vi "navX Open.vi"(4 "Nav6Mode (YPR)":T2, 5 "I2C Bus":T9=enum."I2C MXP", 6 "Serial Port":T1, 7 "SPI Bus":T7=enum."SPI MXP", 8 "error in":errorcluster, 10 "Update Rate (4Hz-60Hz)":T20=50 min=4 max=60 step=1, 11 "navX Interface Protocol":T4) -> (0 "error out":errorcluster, 1 "Opened?":bool, 3 "navX Device TypeDef":T3={"navX Interface Protocol"=enum."SPI", "navX Interface Protocol TypeDefs"={"SPIDevRef"={"DevStatus"={"status"=FALSE, "code"=0, "source"=""}, "Handle"=0, "Controller"=enum."Controller 1", "SPI Bus"=enum."SPI On-Board, CS0"}, "I2CDevRef"={"DevStatus"={"status"=FALSE, "code"=0, "source"=""}, "Controller"=enum."Controller 1", "Device Address"=0, "Handle"=0, "I2C Bus"=enum."Invalid"}, "SerialPortRef"={"DevStatus"={"status"=FALSE, "code"=0, "source"=""}, "Serial Port Name"=""}}, "navX System Information"={"Board Information"={"WhoAmI (50 | 0x32)"=0, "Board Revision"=0, "Firmware Major Version"=0, "Firmware Minor Version"=0, "NAVX_BOARD_CAPABILITY"={"OMNIMOUNT"=FALSE, "YAW_RESET"=FALSE, "VEL_AND_DISP"=FALSE}, "NAVX_BOARD_YAW_AXIS"={"BOARD_YAW_AXIS_UP"=FALSE, "BOARD_YAW_AXIS"=0}}, "Status"={"Update Rate Hz"=0, "Accelerometer Full-Scale Range"=0, "Gyro Full-Scale Range"=0, "NAVX_OP_STATUS"=0, "NAVX_CAL_STATUS"=0, "NAVX_SELFTEST_STATUS"=0, "NAVX_SENSOR_STATUS"={"MOVING"=FALSE, "YAW_STABLE"=FALSE, "MAG_DISTURBANCE"=FALSE, "ALTITUDE_VALID"=FALSE, "SEALEVEL_PRESS_SET"=FALSE, "FUSED_HEADING_VALID"=FALSE}}, "Offsets"={"Yaw"=0.0, "Quat W"=0.0, "Quat X"=0.0, "Quat Y"=0.0, "Quat Z"=0.0}, "LastSampleTimestamp"=0.0, "LastSampleValid"=FALSE}, "navX Common Information"={"Update Rate (4Hz-60Hz)"=50, "refnum name"="", "error"={"status"=FALSE, "code"=0, "source"=""}, "LastFPGATimestamp"=0.0, "Reboot Detected"=FALSE}, "Serial Protocol Extra"={"Loop VI Refnum"=refnum, "Nav6Mode (YPR)"=enum."Raw"}} {"navX Common Information"."Update Rate (4Hz-60Hz)" min=4 max=60 step=1; "navX System Information"."Status"."NAVX_OP_STATUS" items=["INITIALIZING", "SELFTEST_IN_PROGRESS", "ERROR", "IMU_AUTOCAL_IN_PROGRESS", "NORMAL"]; "navX System Information"."Status"."NAVX_CAL_STATUS" items=["IMU_CAL_STATE_MASK"=3, "IMU_CAL_INPROGRESS"=0, "IMU_CAL_ACCUMULATE"=1, "IMU_CAL_COMPLETE"=2, "MAG_CAL_COMPLETE"=4, "BARO_CAL_COMPLETE"=8]; "navX System Information"."Status"."NAVX_SELFTEST_STATUS" items=["COMPLETE"=80, "GYRO_PASSED"=1, "ACCEL_PASSED"=2, "MAG_PASSED"=4, "BARO_PASSED"=8]; "navX Interface Protocol TypeDefs"."I2CDevRef"."Device Address" format="%.0x"})   [LabVIEW 2014, in "navX Library v1 (deprecated).lvlib"]
doc: "This VI is used to open the connection to a navX MXP unit over SPI or I2C."
uses:
  navX Library v1 (deprecated).lvlib
  TypeDefs/Value TypeDefs/navX Interface Protocol.ctl
  TypeDefs/Value TypeDefs/navX Update Rate.ctl
  <vilib>/Rock Robotics/SystemInterfaces/spilib/spi_bus.ctl
  <vilib>/Rock Robotics/SystemInterfaces/i2clib/i2c_bus.ctl
  TypeDefs/navX Device TypeDef.ctl
  <vilib>/Rock Robotics/WPI/SPI/WPI_SPIDevRef.ctl
  <vilib>/Rock Robotics/SystemInterfaces/Typedef/FPGA_TypedefDigitalModule.ctl
  <vilib>/Rock Robotics/WPI/I2C/WPI_I2CDevRef.ctl
  <vilib>/Rock Robotics/WPI/SerialPort/WPI_SerialPortRef.ctl
  TypeDefs/Data TypeDefs/navX Board Information.ctl
  TypeDefs/Value TypeDefs/navX NAVX_BOARD_CAPABILITY.ctl
  TypeDefs/Value TypeDefs/navX NAVX_BOARD_YAW_AXIS.ctl
  TypeDefs/Data TypeDefs/navX Status Data.ctl
  TypeDefs/Value TypeDefs/navX NAVX_OP_STATUS.ctl
  TypeDefs/Value TypeDefs/navX NAVX_CAL_STATUS.ctl
  TypeDefs/Value TypeDefs/navX NAVX_SELFTEST_STATUS.ctl
  TypeDefs/Value TypeDefs/navX NAVX_SENSOR_STATUS.ctl
  TypeDefs/Data TypeDefs/navX Offsets Data.ctl
  TypeDefs/Value TypeDefs/navX Serial Mode.ctl
  NI WPI/WPI_SerialPort_USB.ctl
  TypeDefs/Value TypeDefs/navX Device Registers.ctl
  <vilib>/Rock Robotics/SystemInterfaces/NetworkCommunication/NetComm_UsageReport_ResourceType.ctl
  NI WPI/NI WPI Serial USB.lvlib
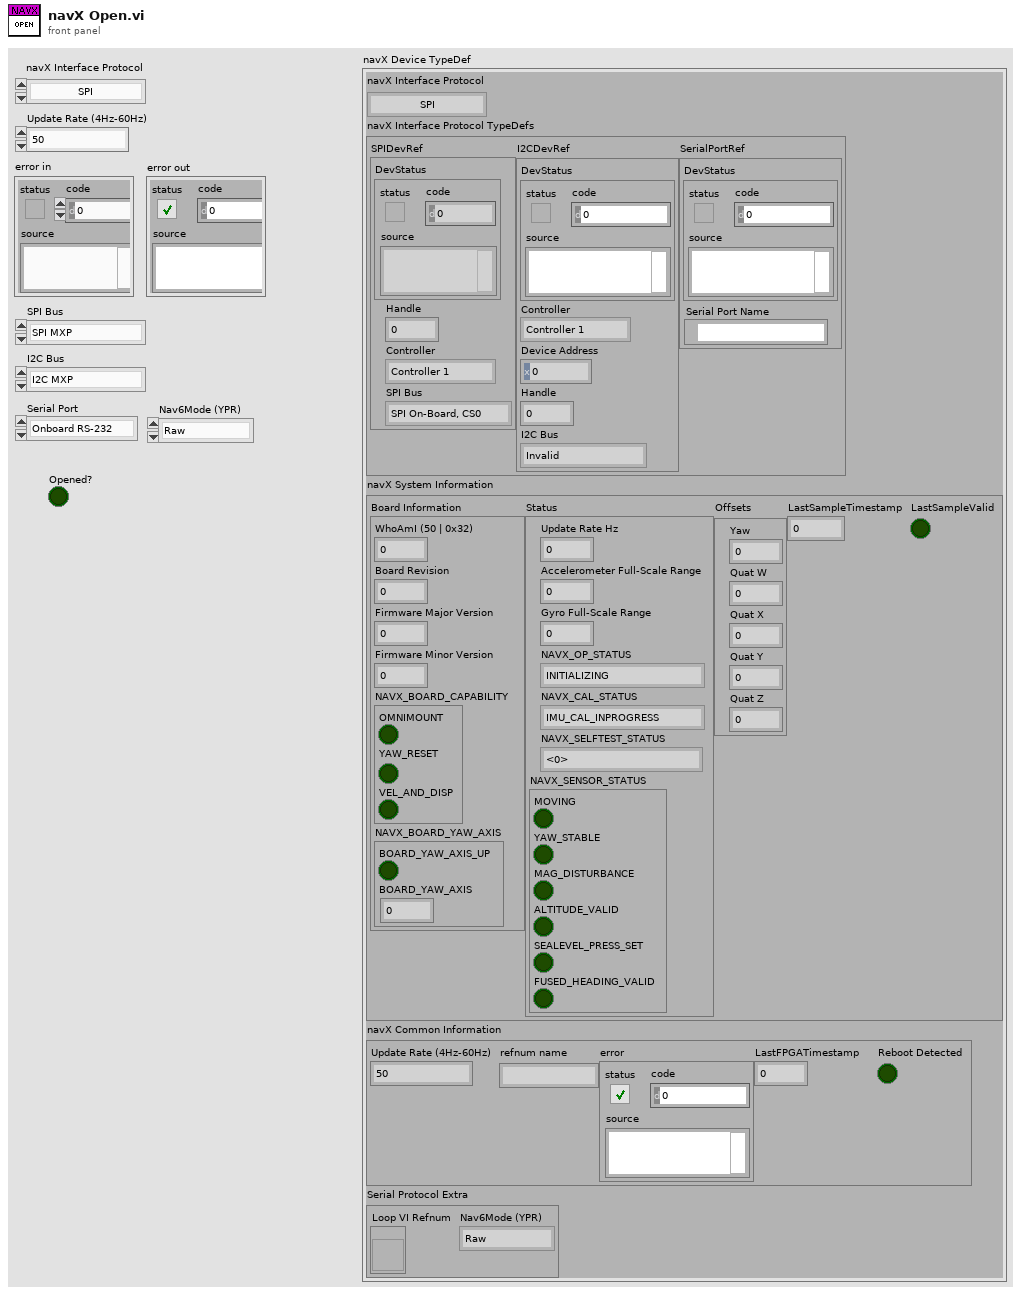
[diagram p1: front panel]
types:
  T1 = typedef "NI WPI Serial USB.lvlib/WPI_SerialPort_USB.ctl" = enum16{"Onboard RS-232", "MXP TTL", "USB"}
  T2 = typedef "navX Library v1 (deprecated).lvlib/navX Serial Mode.ctl" = enum16{"Raw", "Processed"}
  T3 = typedef "navX Library v1 (deprecated).lvlib/navX Device TypeDef.ctl" = cluster{"navX Interface Protocol":T4, "navX Interface Protocol TypeDefs":cluster{"SPIDevRef":T5, "I2CDevRef":T8, "SerialPortRef":T10}, "navX System Information":cluster{"Board Information":T11, "Status":T14, "Offsets":T19, "LastSampleTimestamp":dbl, "LastSampleValid":bool}, "navX Common Information":cluster{"Update Rate (4Hz-60Hz)":T20, "refnum name":string, "error":errorcluster, "LastFPGATimestamp":dbl, "Reboot Detected":bool}, "Serial Protocol Extra":cluster{"Loop VI Refnum":refnum<vi>, "Nav6Mode (YPR)":T2}}
  T4 = typedef "navX Library v1 (deprecated).lvlib/navX Interface Protocol.ctl" = enum16{"SPI", "I2C", "SERIAL"}
  T5 = typedef "WPI_SPIDevRef.ctl" = cluster{"DevStatus":errorcluster, "Handle":i32, "Controller":T6, "SPI Bus":T7}
  T6 = typedef "FPGA_TypedefDigitalModule.ctl" = enum16{"Controller 1"}
  T7 = typedef "spi_bus.ctl" = enum16{"SPI On-Board, CS0", "SPI On-Board, CS1", "SPI On-Board, CS2", "SPI On-Board, CS3", "SPI MXP", "Invalid"}
  T8 = typedef "WPI_I2CDevRef.ctl" = cluster{"DevStatus":errorcluster, "Controller":T6, "Device Address":u8, "Handle":i32, "I2C Bus":T9}
  T9 = typedef "i2c_bus.ctl" = enum16{"I2C On-Board", "I2C MXP", "Invalid"}
  T10 = typedef "WPI_SerialPortRef.ctl" = cluster{"DevStatus":errorcluster, "Serial Port Name":refnum<visa-resource-name>}
  T11 = typedef "navX Library v1 (deprecated).lvlib/navX Board Information.ctl" = cluster{"WhoAmI (50 | 0x32)":u8, "Board Revision":u8, "Firmware Major Version":u8, "Firmware Minor Version":u8, "NAVX_BOARD_CAPABILITY":T12, "NAVX_BOARD_YAW_AXIS":T13}
  T12 = typedef "navX Library v1 (deprecated).lvlib/navX NAVX_BOARD_CAPABILITY.ctl" = cluster{"OMNIMOUNT":bool, "YAW_RESET":bool, "VEL_AND_DISP":bool}
  T13 = typedef "navX Library v1 (deprecated).lvlib/navX NAVX_BOARD_YAW_AXIS.ctl" = cluster{"BOARD_YAW_AXIS_UP":bool, "BOARD_YAW_AXIS":u8}
  T14 = typedef "navX Library v1 (deprecated).lvlib/navX Status Data.ctl" = cluster{"Update Rate Hz":u8, "Accelerometer Full-Scale Range":u8, "Gyro Full-Scale Range":u16, "NAVX_OP_STATUS":T15, "NAVX_CAL_STATUS":T16, "NAVX_SELFTEST_STATUS":T17, "NAVX_SENSOR_STATUS":T18}
  T15 = typedef "navX Library v1 (deprecated).lvlib/navX NAVX_OP_STATUS.ctl" = u8
  T16 = typedef "navX Library v1 (deprecated).lvlib/navX NAVX_CAL_STATUS.ctl" = u8
  T17 = typedef "navX Library v1 (deprecated).lvlib/navX NAVX_SELFTEST_STATUS.ctl" = u8
  T18 = typedef "navX Library v1 (deprecated).lvlib/navX NAVX_SENSOR_STATUS.ctl" = cluster{"MOVING":bool, "YAW_STABLE":bool, "MAG_DISTURBANCE":bool, "ALTITUDE_VALID":bool, "SEALEVEL_PRESS_SET":bool, "FUSED_HEADING_VALID":bool}
  T19 = typedef "navX Library v1 (deprecated).lvlib/navX Offsets Data.ctl" = cluster{"Yaw":dbl, "Quat W":dbl, "Quat X":dbl, "Quat Y":dbl, "Quat Z":dbl}
  T20 = typedef "navX Library v1 (deprecated).lvlib/navX Update Rate.ctl" = u8
  T21 = typedef "navX Library v1 (deprecated).lvlib/navX Device Registers.ctl" = u8
  T22 = typedef "NetComm_UsageReport_ResourceType.ctl" = enum8{"Controller", "Module", "Language", "CANPlugin", "Accelerometer", "ADXL345", "AnalogChannel", "AnalogTrigger", "AnalogTriggerOutput", "CANJaguar", "Compressor", "Counter", "Dashboard", "DigitalInput", "DigitalOutput", "DriverStationCIO", "DriverStationEIO", "DriverStationLCD", "Encoder", "GearTooth", "Gyro", "I2C", "Framework", "Jaguar", "Joystick", "Kinect", "KinectStick", "PIDController", "Preferences", "PWM", "Relay", "RobotDrive", "SerialPort", "Servo", "Solenoid", "SPI", "Task", "Ultrasonic", "Victor", "Button", "Command", "AxisCamera", "PCVideoServer", "SmartDashboard", "Talon", "HiTechnicColorSensor", "HiTechnicAccel", "HiTechnicCompass", "SRF08", "AnalogOutput", "Victor SP", "Talon SRX", "CAN Talon SRX"}
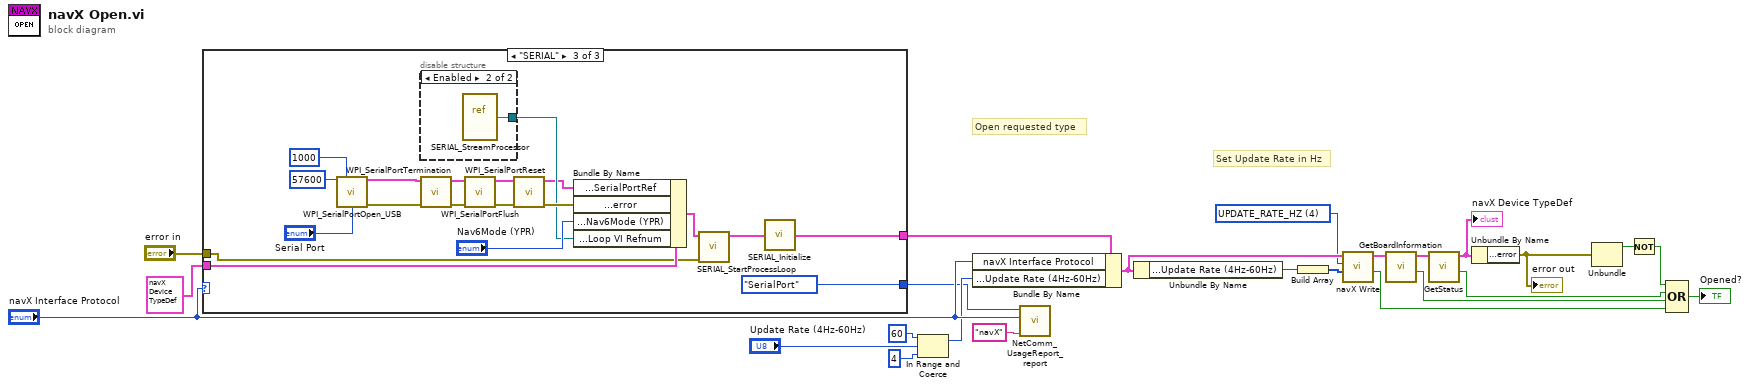
[diagram p0: block diagram]
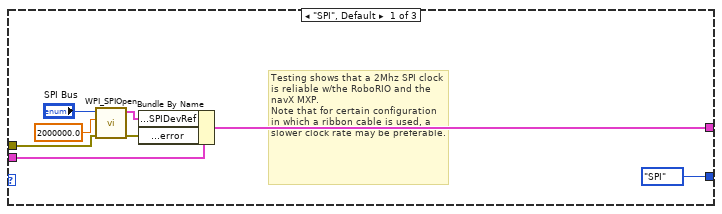
[diagram p2: hidden frame]
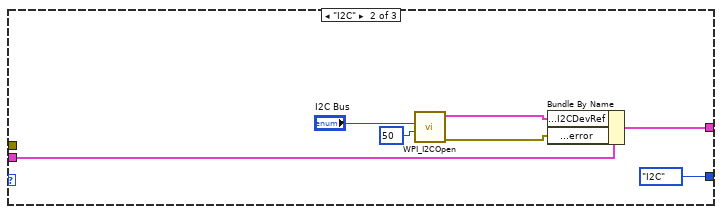
[diagram p3: hidden frame]
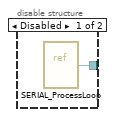
[diagram p4: hidden frame]
diagram:
  w7 = T21 4 items=["WHOAMI"=0, "HW_REV"=1, "FW_VER_MAJOR"=2, "FW_VER_MINOR"=3, "UPDATE_RATE_HZ"=4, "ACCEL_FSR_G"=5, "GYRO_FSR_DPS"=6, "OP_STATUS"=8, "CAL_STATUS"=9, "SELFTEST_STATUS"=10, "SENSOR_STATUS"=16, "TIMESTAMP"=18, "YAW"=22, "PITCH"=24, "ROLL"=26, "HEADING"=28, "FUSED_HEADING"=30, "ALTITUDE_I"=32, "ALTITUDE_D"=34, "LINERA_ACC_X"=36, "LINERA_ACC_Y"=38, "LINERA_ACC_Z"=40, "QUAT_W"=42, "QUAT_X"=44, "QUAT_Y"=46, "QUAT_Z"=48, "MPU_TEMP_C"=50, "GYRO_X"=52, "GYRO_Y"=54, "GYRO_Z"=56, "ACC_X"=58, "ACC_Y"=60, "ACC_Z"=62, "MAG_X"=64, "MAG_Y"=66, "MAG_Z"=68, "PRESSURE_I"=70, "PRESSURE_D"=72, "PRESSURE_TEMP"=74, "YAW_OFFSET"=76, "QUAT_OFFSET_W"=78, "QUAT_OFFSET_X"=80, "QUAT_OFFSET_Y"=82, "QUAT_OFFSET_Z"=84] ("Device Register")
  # "Set Update Rate in Hz"
  # "Open requested type"
  n1 = case shown="\"SERIAL\"" "navX Interface Protocol" {
    tunnel: T3 {"navX Interface Protocol"=enum."SPI", "navX Interface Protocol TypeDefs"={"SPIDevRef"={"DevStatus"={"status"=FALSE, "code"=0, "source"=""}, "Handle"=0, "Controller"=enum."Controller 1", "SPI Bus"=enum."SPI On-Board, CS0"}, "I2CDevRef"={"DevStatus"={"status"=FALSE, "code"=0, "source"=""}, "Controller"=enum."Controller 1", "Device Address"=0, "Handle"=0, "I2C Bus"=enum."Invalid"}, "SerialPortRef"={"DevStatus"={"status"=FALSE, "code"=0, "source"=""}, "Serial Port Name"=""}}, "navX System Information"={"Board Information"={"WhoAmI (50 | 0x32)"=0, "Board Revision"=0, "Firmware Major Version"=0, "Firmware Minor Version"=0, "NAVX_BOARD_CAPABILITY"={"OMNIMOUNT"=FALSE, "YAW_RESET"=FALSE, "VEL_AND_DISP"=FALSE}, "NAVX_BOARD_YAW_AXIS"={"BOARD_YAW_AXIS_UP"=FALSE, "BOARD_YAW_AXIS"=0}}, "Status"={"Update Rate Hz"=0, "Accelerometer Full-Scale Range"=0, "Gyro Full-Scale Range"=0, "NAVX_OP_STATUS"=0, "NAVX_CAL_STATUS"=0, "NAVX_SELFTEST_STATUS"=0, "NAVX_SENSOR_STATUS"={"MOVING"=FALSE, "YAW_STABLE"=FALSE, "MAG_DISTURBANCE"=FALSE, "ALTITUDE_VALID"=FALSE, "SEALEVEL_PRESS_SET"=FALSE, "FUSED_HEADING_VALID"=FALSE}}, "Offsets"={"Yaw"=0.0, "Quat W"=0.0, "Quat X"=0.0, "Quat Y"=0.0, "Quat Z"=0.0}, "LastSampleTimestamp"=0.0, "LastSampleValid"=FALSE}, "navX Common Information"={"Update Rate (4Hz-60Hz)"=50, "refnum name"="", "error"={"status"=FALSE, "code"=0, "source"=""}, "LastFPGATimestamp"=0.0, "Reboot Detected"=FALSE}, "Serial Protocol Extra"={"Loop VI Refnum"=refnum, "Nav6Mode (YPR)"=enum."Raw"}} ("navX Device TypeDef") -> [w32 w39 w58]
    tunnel: [w29 w38 w41] -> w10
    tunnel: "error in" -> [w28 _ w44]
    tunnel: [NetComm_UsageReport_ResourceType."SPI" ("Resource Type") NetComm_UsageReport_ResourceType."I2C" ("Resource Type") NetComm_UsageReport_ResourceType."SerialPort" ("Resource Type")] -> w9
    frame "SPI", Default {
      # "Testing shows that a 2Mhz SPI clock is reliable w/the RoboRIO and the navX MXP. \nNote that for certain configuration in which a ribbon cable is used, a slower clock rate may be preferable."
      n2 = call <vilib>:"WPI_SPIOpen.vi"("error in"=w28, "Clock Rate (Hz)"=2000000.0, "SPI Bus"="SPI Bus") -> ("error out"=w31:errorcluster, "SPIDevRef"=w30:T5)  [unwired: 7 in]
      n3 = Bundle By Name(cluster=w32, "navX Interface Protocol TypeDefs.SPIDevRef"=w30, "navX Common Information.error"=w31) -> (w29:T3)
    }
    frame "I2C" {
      n4 = call <vilib>:"WPI_I2COpen.vi"("Device Address"=u8 50, "I2C Bus"="I2C Bus") -> ("error out"=w37:errorcluster, "I2CDevRef"=w36:T8)  [unwired: 8 in]
      n5 = Bundle By Name(cluster=w39, "navX Interface Protocol TypeDefs.I2CDevRef"=w36, "navX Common Information.error"=w37) -> (w38:T3)
    }
    frame "SERIAL" {
      n6 = call "WPI_SerialPortOpen_USB.vi"("Baud Rate"=u32 57600, "Timeout Value (ms)"=u32 1000, "Serial Port"="Serial Port") -> ("SerialPortRef"=w56:T10, "error out"=w57:errorcluster)  [unwired: 11 in]
      n7 = disable-structure shown="Enabled" {
        disable-tunnel: [w59 w60] -> w46
        frame Disabled {
          n8 = vi-ref "SERIAL_ProcessLoop.vi"() -> (w59:refnum<vi>)
        }
        frame Enabled {
          n9 = vi-ref "SERIAL_StreamProcessor.vi"() -> (w60:refnum<vi>)
        }
      }
      n10 = call <vilib>:"WPI_SerialPortTermination.vi"("error in (no error)"=w57, "SerialPortRef"=w56) -> ("error out"=w53:errorcluster, "SerialPortRef"=w52:T10)  [unwired: 8 in]
      n11 = call <vilib>:"WPI_SerialPortFlush.vi"("error in (no error)"=w53, "SerialPortRef"=w52) -> ("error out"=w50:errorcluster, "SerialPortRef"=w51:T10)  [unwired: 8 in]
      n12 = call <vilib>:"WPI_SerialPortReset.vi"("error in (no error)"=w50, "SerialPortRef"=w51) -> ("error out"=w49:errorcluster, "SerialPortRef"=w45:T10)  [unwired: 8 in]
      n13 = Bundle By Name(cluster=w58, "navX Interface Protocol TypeDefs.SerialPortRef"=w45, "navX Common Information.error"=w49, "Serial Protocol Extra.Nav6Mode (YPR)"="Nav6Mode (YPR)", "Serial Protocol Extra.Loop VI Refnum"=w46) -> (w43:T3)
      n14 = call "SERIAL_StartProcessLoop.vi"("error in (no error)"=w44, "navX Device TypeDef"=w43) -> ("navX Device TypeDef"=w42:T3)  [unwired: 8 in, 1 out]
      n15 = call "SERIAL_Initialize.vi"("navX Device TypeDef"=w42) -> ("navX Device TypeDef"=w41:T3)
    }
  }
  n16 = In Range and Coerce(upper limit=u8 60, x="Update Rate (4Hz-60Hz)", lower limit=u8 4) -> (coerced(x)=w17:T20)  [unwired: 1 out]
  n17 = Bundle By Name(cluster=w10, "navX Interface Protocol"="navX Interface Protocol", "navX Common Information.Update Rate (4Hz-60Hz)"=w17) -> (w21:T3)
  n18 = call <vilib>:"NetComm_UsageReport_report.vi"("Feature"="navX", "Instance Number"="navX Interface Protocol", "Resource Type"=w9) -> ()  [unwired: 9 in]
  n19 = Unbundle By Name(w21) -> ("navX Common Information.Update Rate (4Hz-60Hz)"=w6:T20)
  n20 = Build Array(w6) -> (w5:T20[])
  n21 = call "navX Write.vi"("navX Message"=w5, "Device Register"=w7, "navX Device TypeDef"=w21) -> ("Valid?"=w11:bool, "navX Device TypeDef"=w16:T3)  [unwired: 7 in]
  n22 = call "GetBoardInformation.vi"("navX Device TypeDef"=w16) -> ("Valid?"=w15:bool, "navX Device TypeDef"=w4:T3)  [unwired: 8 in, 1 out]
  n23 = call "GetStatus.vi"("navX Device TypeDef"=w4) -> ("Valid?"=w14:bool, "navX Device TypeDef"=w13:T3)  [unwired: 8 in, 1 out]
  "navX Device TypeDef" <- w13
  n24 = Unbundle By Name(w13) -> ("navX Common Information.error"=w3:errorcluster)
  "error out" <- w3
  n25 = Unbundle(w3) -> ("status"=w2:bool)  [unwired: 2 out]
  n26 = Not(x=w2) -> (.not. x?=w1:bool)
  n27 = Compound Arithmetic op=OR(w1, w14, w15, w11) -> (→"Opened?":bool)
